vi "Position Shutdown Button.vi"(8 "error in (no error)":errorcluster, 10 "Previous Button Refnum":refnum<vi>, 11 "Shutdon Button":refnum<vi>) -> (0 "error out":errorcluster)   [LabVIEW 2014]
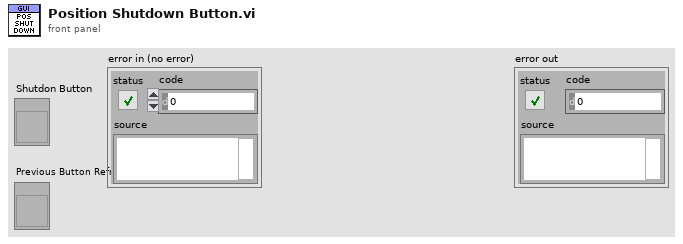
[diagram p1: front panel]
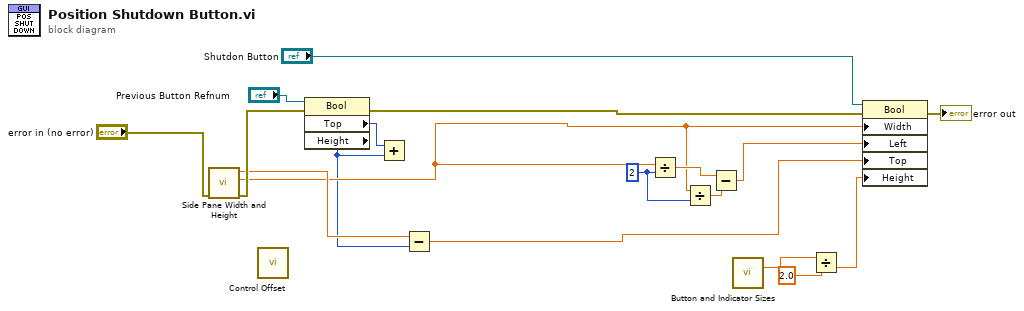
[diagram p0: block diagram]
diagram:
  w14 = u32 2 ("y")
  n1 = call "Side Pane Width and Height.vi"("error in (no error)"="error in (no error)") -> ("error out"=w9:errorcluster, "Width"=w3:dbl, "Height"=w4:dbl)  [unwired: 8 in]
  n2 = call "Control Offset.vi"() -> ()  [unwired: 11 in, 1 out]
  n3 = property class="Bool"(reference="Previous Button Refnum", error in=w9) -> (error out=w16:errorcluster, "Top"=w8:i32, "Height"=w1:u32)  [unwired: 1 out]
  n4 = Add(x=w8, y=w1) -> ()  [unwired: 1 out]
  n5 = Subtract(x=w4, y=w1) -> (x-y=w2:dbl)
  n6 = Divide(x=w3, y=w14) -> (x/y=w15:dbl)
  n7 = Divide(x=w3, y=w14) -> (x/y=w13:dbl)
  n8 = Subtract(x=w15, y=w13) -> (x-y=w12:dbl)
  n9 = call "Button and Indicator Sizes.vi"() -> ("Button Height"=w6:dbl)  [unwired: 11 in, 4 out]
  n10 = Divide(x=w6, y=2.0) -> (x/y=w7:dbl)
  n11 = property class="Bool"(reference="Shutdon Button", error in=w16, "Width"=w3, "Left"=w12, "Top"=w2, "Height"=w7) -> (error out=→"error out":errorcluster)  [unwired: 1 out]
